vi "Periodic Random Noise PtByPt.vi"(2 "initialize":bool, 3 "seed":i32=-1, 4 "spectral amplitude":dbl=1.0 format="%0.2f", 5 "sample length":i32=100) -> (0 "error":i32, 1 "periodic random noise":dbl format="%0.2f")   [LabVIEW 2020, in "NI_PtbyPt.lvlib"]
doc: "Generates a set of output data that contains periodic random noise (PRN)."
uses:
  NI_PtbyPt.lvlib
  NI_AALBase.lvlib
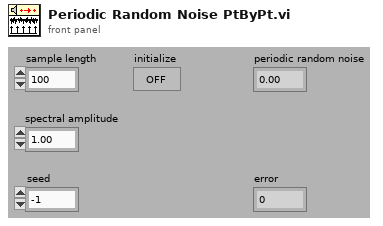
[diagram p1: front panel]
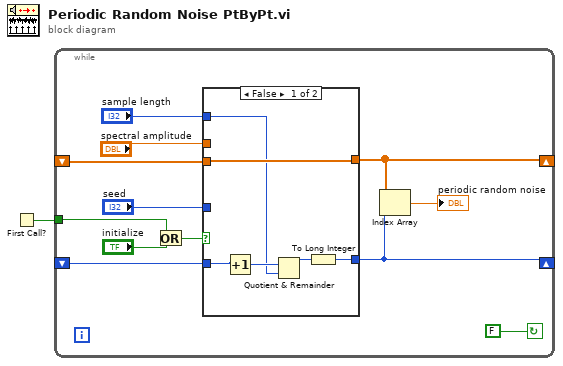
[diagram p0: block diagram]
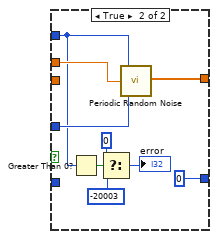
[diagram p2: hidden frame]
diagram:
  n1 = First Call?() -> (First Call?: T/F=w1:bool)
  n2 = while {
    tunnel: w1 -> [w4]
    shift-left: _ -> [w7]
    shift-right: [w6] -> _
    shift-left: _ -> [w9]
    shift-right: [w11] -> _
    stop <- FALSE continue-if-true
    n3 = Or(x=w4, y="initialize") -> (x .or. y?=w3:bool)
    n4 = case shown="False" w3 {
      tunnel: "sample length" -> [w16 w23]
      tunnel: "spectral amplitude" -> [_ w28]
      tunnel: "seed" -> [_ w27]
      tunnel: [w19 w26] -> w11
      tunnel: w9 -> [w19 _]
      tunnel: [w14 0] -> w6
      tunnel: w7 -> [w18 _]
      frame False {
        n5 = Increment(x=w18) -> (x+1=w17:i32)
        n6 = Quotient & Remainder(x=w17, y=w16) -> (x-y*floor(x/y)=w15:i32)  [unwired: 1 out]
        n7 = To Long Integer(number=w15) -> (32bit integer=w14:i32)
      }
      frame True {
        n8 = Greater Than 0?(x=w23) -> (x > 0?=w24:bool)
        n9 = Select(t=0, s=w24, f=-20003) -> (s? t:f=→"error":i32)
        n10 = call "Periodic Random Noise.vi"("seed"=w27, "spectral amplitude"=w28, "samples"=w23) -> ("periodic random noise"=w26:dbl[])  [unwired: 1 out]
      }
    }
    n11 = Index Array(array=w11, index=w6) -> (element=→"periodic random noise":dbl)
  }
